vi "PathPlanner_Trajectory_RecalculateValues.vi"(9 "Reversed":bool, 11 "PathPlannerStates":T1[](array[typedef]) {"TargetHolonomicRotation"."SIN" format="%13.4f"; "TargetHolonomicRotation"."COS" format="%13.4f"; "TargetHolonomicRotation"."VALUE" format="%13.4f"; "Heading"."SIN" format="%13.4f"; "Heading"."COS" format="%13.4f"; "Heading"."VALUE" format="%13.4f"; "PositionMeters"."Y" format="%14.3f"; "PositionMeters"."X" format="%14.3f"}) -> (3 "outPathPlannerStates":T1[](array[typedef]) {"TargetHolonomicRotation"."SIN" format="%13.4f"; "TargetHolonomicRotation"."COS" format="%13.4f"; "TargetHolonomicRotation"."VALUE" format="%13.4f"; "Heading"."SIN" format="%13.4f"; "Heading"."COS" format="%13.4f"; "Heading"."VALUE" format="%13.4f"; "PositionMeters"."Y" format="%14.3f"; "PositionMeters"."X" format="%14.3f"})   [LabVIEW 2019, in "PathPlanner24.lvlib"]
uses:
  PathPlanner24.lvlib
  <vilib>/Rock Robotics/WPI/ThirdParty/JAS_Junk/TrajLib/Trajectory_Library.lvlib
  <vilib>/Rock Robotics/WPI/ThirdParty/JAS_Junk/TrajLib/TypeDef/ROTATION2D.ctl
  <vilib>/Rock Robotics/WPI/ThirdParty/JAS_Junk/TrajLib/TypeDef/TRANSLATION2D.ctl
  TypeDef/PathPlannerTrajectoryState.ctl
  TypeDef/PathPlannerConstraints.ctl
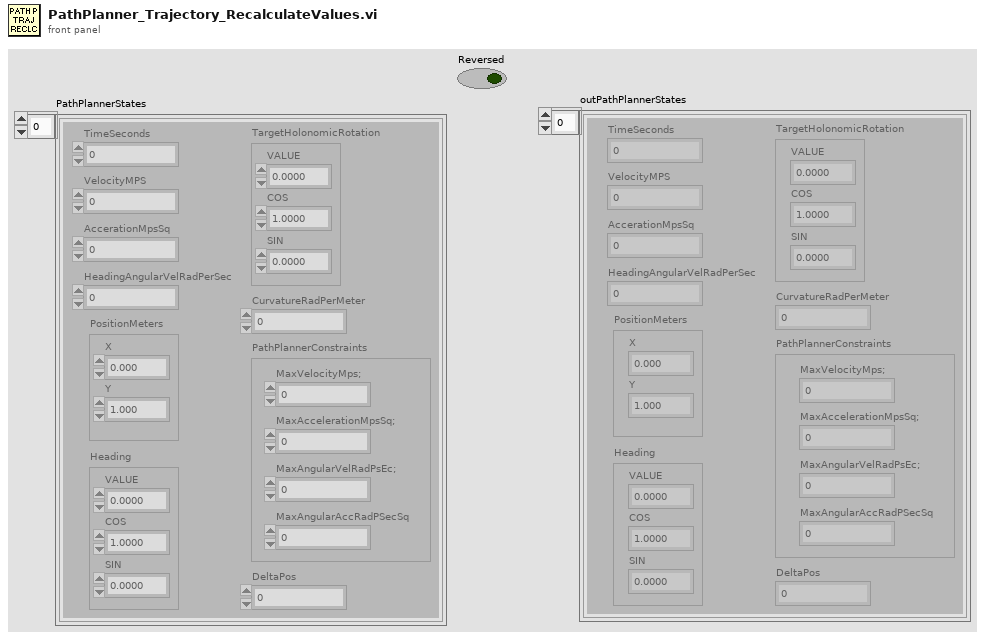
[diagram p1: front panel]
types:
  T1 = typedef "PathPlanner24.lvlib/PathPlannerTrajectoryState.ctl" = cluster{"TimeSeconds":dbl, "VelocityMPS":dbl, "AccerationMpsSq":dbl, "HeadingAngularVelRadPerSec":dbl, "PositionMeters":T2, "Heading":T3, "TargetHolonomicRotation":T3, "CurvatureRadPerMeter":dbl, "DeltaPos":dbl, "PathPlannerConstraints":T4}
  T2 = typedef "Trajectory_Library.lvlib/TRANSLATION2D.ctl" = cluster{"X":dbl, "Y":dbl}
  T3 = typedef "Trajectory_Library.lvlib/ROTATION2D.ctl" = cluster{"VALUE":dbl, "COS":dbl, "SIN":dbl}
  T4 = typedef "PathPlanner24.lvlib/PathPlannerConstraints.ctl" = cluster{"MaxVelocityMps;":dbl, "MaxAccelerationMpsSq;":dbl, "MaxAngularVelRadPsEc;":dbl, "MaxAngularAccRadPSecSq":dbl}
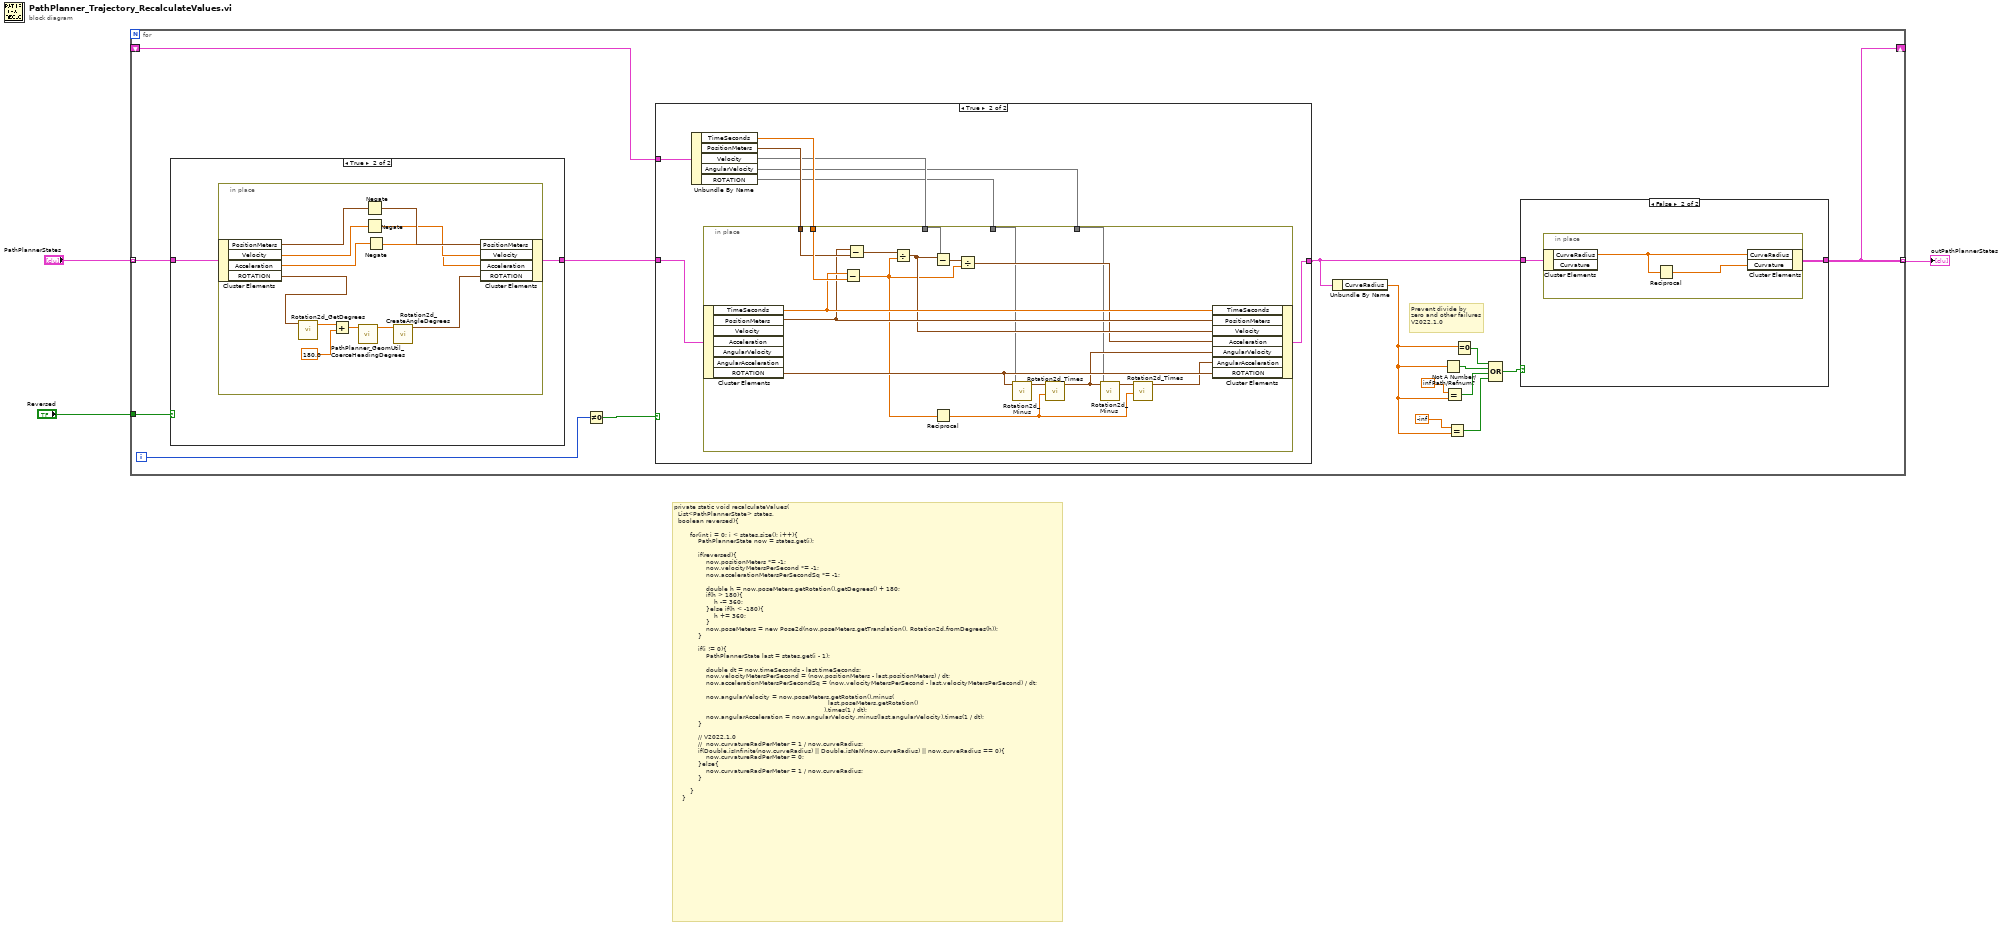
[diagram p0: block diagram]
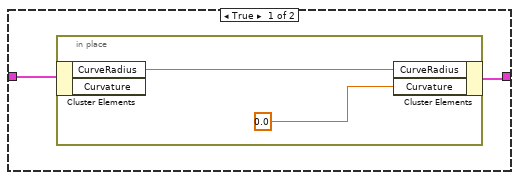
[diagram p2: hidden frame]
diagram:
  # "private static void recalculateValues(\n\t\tList<PathPlannerState> states, \n\t\tboolean reversed){\n\n        for(int i = 0; i < states.size(); i++){\n            PathPlannerState now = states.get(i);\n\n            if(reversed){\n                now.positionMeters *= -1;\n                now.velocityMetersPerSecond *= -1;\n                now.accelerationMetersPerSecondSq *= -1;\n\n                double h = now.poseMeters.getRotation().getDegrees() + 180;\n                if(h > 180){\n                    h -= 360;\n                }else if(h < -180){\n                    h += 360;\n                }\n                now.poseMeters = new Pose2d(now.poseMeters.getTranslation(), Rotation2d.fromDegrees(h));\n            }\n\n            if(i != 0){\n                PathPlannerState last = states.get(i - 1);\n\n                double dt = now.timeSeconds - last.timeSeconds;\n                now.velocityMetersPerSecond = (now.positionMeters - last.positionMeters) / dt;\n                now.accelerationMetersPerSecondSq = (now.velocityMetersPerSecond - last.velocityMetersPerSecond) / dt;\n\n                now.angularVelocity = now.poseMeters.getRotation().minus(\n\t\t\t\t                                                                         last.poseMeters.getRotation()\n                                                                           ).times(1 / dt);\n                now.angularAcceleration = now.angularVelocity.minus(last.angularVelocity).times(1 / dt);\n            }\n\n            // V2022.1.0\n            //  now.curvatureRadPerMeter = 1 / now.curveRadius;   \n            if(Double.isInfinite(now.curveRadius) || Double.isNaN(now.curveRadius) || now.curveRadius == 0){\n                now.curvatureRadPerMeter = 0;\n            }else{\n                now.curvatureRadPerMeter = 1 / now.curveRadius;\n            }\n \n        }\n    }"
  n1 = for {
    tunnel: "PathPlannerStates" -> [w18] mode=indexing
    tunnel: "Reversed" -> [w19]
    tunnel: [w13] -> w1 mode=indexing
    shift-right: [w13] -> _
    shift-left: _ -> [w14]
    i -> [w17]
    # "Prevent divide by\nzero and other failures\nV2022.1.0"
    n2 = case shown="True" w19 {
      tunnel: w18 -> [w55 w57]
      tunnel: [w55 w56] -> w15
      frame False {
      }
      frame True {
        n3 = in-place {
          n4 = in-place-cluster #1(w57) -> ("PositionMeters"=w69:T2, "Velocity"=w67:dbl, "Acceleration"=w65:dbl, "ROTATION"=w59:T3)
          n5 = call <vilib>:"Rotation2d_GetDegrees.vi"("in ROTATION"=w59) -> ("AngleDegrees"=w58:dbl)  [unwired: 10 in]
          n6 = Add(x=w58, y=180.0) -> (x+y=w60:dbl)
          n7 = call "PathPlanner_GeomUtil_CoerceHeadingDegrees.vi"("in Degrees"=w60) -> ("out Degrees"=w61:dbl)  [unwired: 10 in]
          n8 = Negate(x=w69) -> (-x=w68:T2)
          n9 = Negate(x=w67) -> (-x=w66:dbl)
          n10 = Negate(x=w65) -> (-x=w64:dbl)
          n11 = call <vilib>:"Rotation2d_CreateAngleDegrees.vi"("Angle_Degrees"=w61) -> ("ROTATION"=w62:T3)  [unwired: 10 in]
          n12 = in-place-cluster #1("PositionMeters"=w68, "Velocity"=w66, "Acceleration"=w64, "ROTATION"=w62) -> (w56:T1)
        }
      }
    }
    n13 = Not Equal To 0?(x=w17) -> (x != 0?=w16:bool)
    n14 = case shown="True" w16 {
      tunnel: w15 -> [w28 w36]
      tunnel: [w28 w29] -> w12
      tunnel: w14 -> [_ w35]
      frame False {
      }
      frame True {
        n15 = Unbundle By Name(w35) -> ("TimeSeconds"=w34:dbl, "PositionMeters"=w33:T2, "Velocity"=w32, "AngularVelocity"=w30, "ROTATION"=w31)
        n16 = in-place {
          in-place-border: w34 -> [w54]
          in-place-border: w33 -> [w53]
          in-place-border: w32 -> [w49]
          in-place-border: w31 -> [w44]
          in-place-border: w30 -> [w40]
          n17 = in-place-cluster #2(w36) -> ("TimeSeconds"=w52:dbl, "PositionMeters"=w51:T2, "ROTATION"=w45:T3)  [unwired: 4 out]
          n18 = Subtract(x=w52, y=w54) -> (x-y=w38:dbl)
          n19 = Subtract(x=w51, y=w53) -> (x-y=w39:T2)
          n20 = Divide(x=w39, y=w38) -> (x/y=w50:T2)
          n21 = Subtract(x=w50, y=w49) -> (x-y=w48:T2)
          n22 = Reciprocal(x=w38) -> (1/x=w37:dbl)
          n23 = Divide(x=w48, y=w38) -> (x/y=w47:T2)
          n24 = call <vilib>:"Rotation2d_Minus.vi"("other ROTATION"=w44, "in ROTATION"=w45) -> ("out ROTATION"=w46:T3)  [unwired: 9 in]
          n25 = call <vilib>:"Rotation2d_Times.vi"("Scalar"=w37, "in ROTATION"=w46) -> ("out ROTATION"=w42:T3)  [unwired: 9 in]
          n26 = call <vilib>:"Rotation2d_Minus.vi"("other ROTATION"=w40, "in ROTATION"=w42) -> ("out ROTATION"=w43:T3)  [unwired: 9 in]
          n27 = call <vilib>:"Rotation2d_Times.vi"("Scalar"=w37, "in ROTATION"=w43) -> ("out ROTATION"=w41:T3)  [unwired: 9 in]
          n28 = in-place-cluster #2("TimeSeconds"=w52, "PositionMeters"=w51, "Velocity"=w50, "Acceleration"=w47, "AngularVelocity"=w42, "AngularAcceleration"=w41, "ROTATION"=w45) -> (w29:T1)
        }
      }
    }
    n29 = Unbundle By Name(w12) -> ("CurveRadius"=w8:dbl)
    n30 = Not A Number/Path/Refnum?(number/path/refnum=w8) -> (NaN/Path/Refnum?=w6:bool)
    n31 = Equal?(x=inf, y=w8) -> (x = y?=w5:bool)
    n32 = Equal?(x=-inf, y=w8) -> (x = y?=w4:bool)
    n33 = Equal To 0?(x=w8) -> (x = 0?=w10:bool)
    n34 = Compound Arithmetic op=OR(w10, w6, w5, w4) -> (w11:bool)
    n35 = case shown="False" w11 {
      tunnel: w12 -> [w21 w25]
      tunnel: [w20 w24] -> w13
      frame True {
        n36 = in-place {
          n37 = in-place-cluster #3(w21) -> ("CurveRadius"=w23:dbl)  [unwired: 1 out]
          n38 = in-place-cluster #3("CurveRadius"=w23, "Curvature"=0.0 ("TrajectoryState.Curvature")) -> (w20:T1)
        }
      }
      frame False {
        n39 = in-place {
          n40 = in-place-cluster #4(w25) -> ("CurveRadius"=w27:dbl)  [unwired: 1 out]
          n41 = Reciprocal(x=w27) -> (1/x=w26:dbl)
          n42 = in-place-cluster #4("CurveRadius"=w27, "Curvature"=w26) -> (w24:T1)
        }
      }
    }
  }
  "outPathPlannerStates" <- w1
